vi "XY Graph Multiplot Math Window.vi"(8 "Error In":errorcluster, 11 "XY Graph":refnum<vi>) -> (0 "Error Out":errorcluster, 1 "Cancelled":bool, 2 "Plot Destination Output":T2, 3 "Plot Formula Definition output":T1)   [LabVIEW 2021, in "XY Graph Add-Ons.lvlib"]
uses:
  XY Graph Add-Ons.lvlib
  Plot Destination.ctl
  XY Graph Plot Formula Definitiion.ctl
  <vilib>/gmath/NI_Gmath.lvlib
  Graphs.lvlib
panel:
  in  "Plot Formula Definition":T1
  out "Valid formula":bool
  out "Same abscissa array":bool
  in  "Plot Destination":T2=enum."New Plot"
  in  "OK":bool
  in  "Cancel":bool
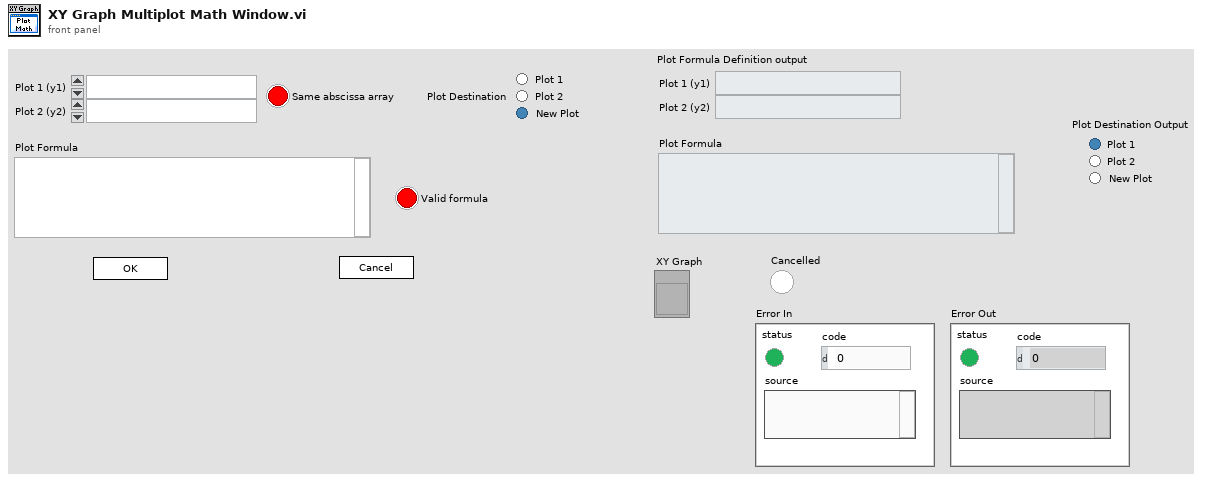
[diagram p1: front panel]
types:
  T1 = typedef "XY Graph Add-Ons.lvlib/XY Graph Plot Formula Definitiion.ctl" = cluster{"Plot 1 (y1)":u16, "Plot 2 (y2)":u16, "Plot Formula":string}
  T2 = typedef "Graphs.lvlib/Plot Destination.ctl" = enum32{"Plot 1", "Plot 2", "New Plot"}
  T3 = typedef "XY Graph Add-Ons.lvlib/XY Graph Refnum.ctl" = refnum<vi>
  T4 = typedef "XY Graph Add-Ons.lvlib/XY Plot Data.ctl" = cluster{"X Array":dbl[], "Y Array":dbl[]}
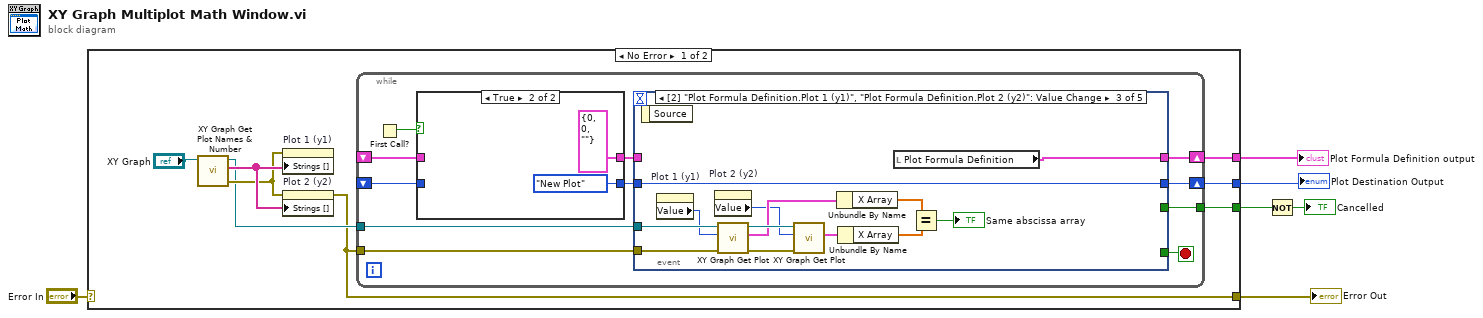
[diagram p0: block diagram]
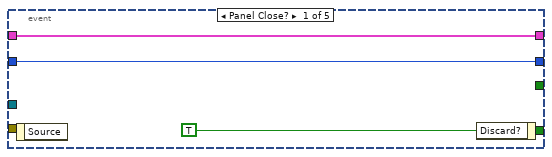
[diagram p3: hidden frame]
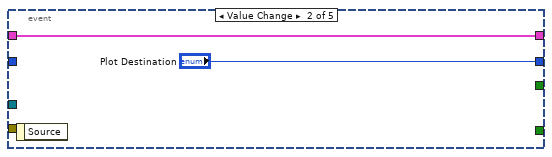
[diagram p4: hidden frame]
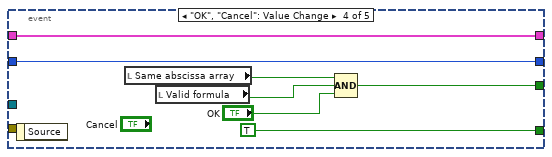
[diagram p5: hidden frame]
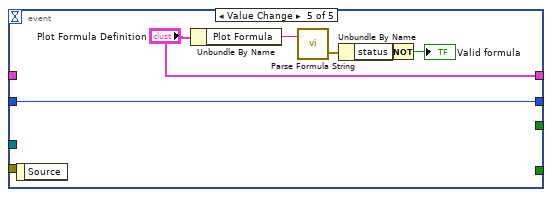
[diagram p6: hidden frame]
diagram:
  n1 = case shown="No Error" "Error In" {
    selector: "Error In" -> [_ w61]
    tunnel: [w14 _] -> w6
    tunnel: [w13 _] -> w2
    tunnel: [w11 _] -> w3
    tunnel: [w7 w61] -> w1
    frame No Error {
      n2 = call "XY Graph Get Plot Names & Number.vi"("XYGraph in"="XY Graph") -> ("error out"=w9:errorcluster, "Plot Names"=w10:string[], "XYGraph out"=w8:T3)  [unwired: 5 in, 3 out]
      n3 = property on="Plot 1 (y1)" class="Ring (strict)"(error in=w9, "Strings []"=w10) -> ()  [unwired: 1 in, 2 out]
      n4 = property on="Plot 2 (y2)" class="Ring (strict)"(error in=w9, "Strings []"=w10) -> (error out=w7:errorcluster)  [unwired: 1 in, 1 out]
      n5 = while {
        tunnel: [w24] -> w14
        shift-right: [w23] -> w13
        shift-left: _ -> [w18]
        shift-right: [w22] -> w11
        shift-left: _ -> [w17]
        tunnel: w8 -> [w21]
        tunnel: w7 -> [w20]
        stop <- w25 stop-if-true
        n6 = First Call?() -> (First Call?: T/F=w19:bool)
        n7 = case shown="True" w19 {
          tunnel: w18 -> [w27 _]
          tunnel: w17 -> [w26 _]
          tunnel: [w27 T1 {"Plot 1 (y1)"=0, "Plot 2 (y2)"=0, "Plot Formula"=""} ("Plot Formula Definition")] -> w16
          tunnel: [w26 Plot_Destination."New Plot" ("Plot Destination")] -> w15
          frame False {
          }
          frame True {
          }
        }
        n8 = event shown="[2] \"Plot Formula Definition.Plot 1 (y1)\", \"Plot Formula Definition.Plot 2 (y2)\": Value Change" {
          selector: _ -> [_ _ _ _ _]
          dyn-events: _ -> [_ _ _ _ _]
          timeout: _ -> [_ _ _ _ _]
          tunnel: [w32 _ _ TRUE ("Discard?") _] -> w25
          tunnel: [_ _ _ w51 _] -> w24
          tunnel: [w31 w33 w37 w53 "Plot Formula Definition"] -> w23
          tunnel: w16 -> [w31 w33 _ w53 _]
          tunnel: [w30 "Plot Destination" w47 w52 w60] -> w22
          tunnel: w15 -> [w30 _ w47 w52 w60]
          tunnel: w21 -> [_ _ w46 _ _]
          tunnel: w20 -> [_ _ w45 _ _]
          event Panel Close? {
            w32 = TRUE ("Discard?")
            n9 = event-data() -> ()  [unwired: 1 in, 1 out]
            n10 = event-data("Discard?"=w32) -> ()  [unwired: 1 in, 1 out]
          }
          event Value Change {
            n11 = event-data() -> ()  [unwired: 1 in, 1 out]
          }
          event Value Change {
            n12 = event-data() -> ()  [unwired: 1 in, 1 out]
            n13 = property on="Plot 1 (y1)" class="Ring (strict)"() -> ("Value"=w36:u16)  [unwired: 2 in, 2 out]
            n14 = property on="Plot 2 (y2)" class="Ring (strict)"() -> ("Value"=w35:u16)  [unwired: 2 in, 2 out]
            n15 = call "XY Graph Get Plot.vi"("error in (no error)"=w45, "Plot Index (-1: last)"=w36, "XYGraph in"=w46) -> ("error out"=w44:errorcluster, "Plot Data"=w42:T4, "XYGraph out"=w43:T3)  [unwired: 4 in, 2 out]
            n16 = call "XY Graph Get Plot.vi"("error in (no error)"=w44, "Plot Index (-1: last)"=w35, "XYGraph in"=w43) -> ("Plot Data"=w41:T4)  [unwired: 4 in, 4 out]
            n17 = Unbundle By Name(w42) -> ("X Array"=w40:dbl[])
            n18 = Unbundle By Name(w41) -> ("X Array"=w39:dbl[])
            n19 = local read "Plot Formula Definition"() -> (w37:T1)
            n20 = Equal?(x=w40, y=w39) -> (x = y?=→"Same abscissa array":bool)
          }
          event "OK", "Cancel": Value Change {
            n21 = event-data() -> ()  [unwired: 1 in, 1 out]
            n22 = local read "Same abscissa array"() -> (w50:bool)
            n23 = local read "Valid formula"() -> (w48:bool)
            n24 = Compound Arithmetic op=AND(w50, w48, "OK") -> (w51:bool)
          }
          event Value Change {
            n25 = event-data() -> ()  [unwired: 1 in, 1 out]
            n26 = Unbundle By Name("Plot Formula Definition") -> ("Plot Formula"=w59:string)
            n27 = call <vilib>:"Parse Formula String.vi"("formula"=w59) -> ("error out"=w58:errorcluster)  [unwired: 1 in, 1 out]
            n28 = Unbundle By Name(w58) -> ("status"=w57:bool)
            n29 = Not(x=w57) -> (.not. x?=→"Valid formula":bool)
          }
        }
      }
    }
    frame Error {
    }
  }
  "Error Out" <- w1
  "Plot Destination Output" <- w3
  "Plot Formula Definition output" <- w2
  n30 = Not(x=w6) -> (.not. x?=→"Cancelled":bool)
